vi "Ex_Inst_Write LabVIEW Measurement File.vi"(0 "Signals":dynamicdata(waveform), 2 "Enable":bool=TRUE, 5 "error in (no error)":errorcluster, 8 "Filename":path, 10 "Comment":string, 11 "DAQmx Task":refnum<k21>) -> (16 "Filename Out":path, 17 "Saving Data":bool, 19 "error out":errorcluster)   [LabVIEW 2020]
doc: "Writes data to text-based measurement files (.lvm), binary measurement files (.tdm or .tdms), or Microsoft Excel files (.xlsx)."
uses:
  <vilib>/express/express shared/ExFile.llb/ex_FileFormats.ctl
  <vilib>/express/express shared/ExFile.llb/ex_userDefProperty.ctl
  <vilib>/express/express shared/ex_EditUserDefinedProperties/usiDataType.ctl
  <vilib>/express/express shared/ExFile.llb/ex_propertySource.ctl
panel:
  in  "Live values":variant[](array[variant])
  in  "new_file":bool
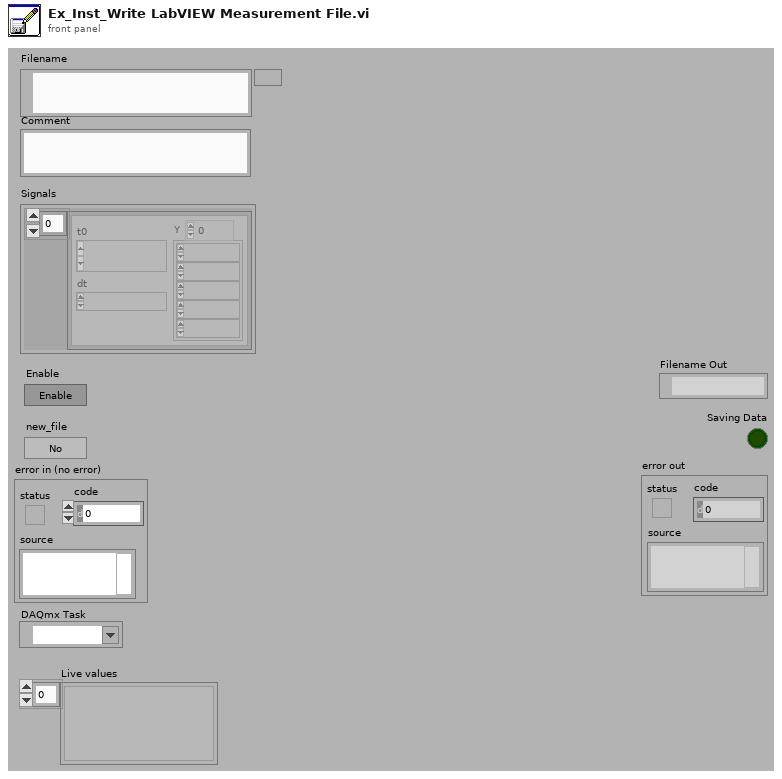
[diagram p1: front panel]
types:
  T1 = cluster{"Boolean":bool, "Timestamp format":string}
  T2 = typedef "ex_FileFormats.ctl" = enum32{"lvm", "tdm", "tdms", "xlsx"}
  T3 = typedef "ex_userDefProperty.ctl" = cluster{"Name":string, "Object type":string, "usiDataType":T4, "propertySourceType":T5, "propertySource":string, "Value":variant, "ID":i32, "use def name":bool, "Source":string, "Built-in Prop":bool, "Attribute Type Enum":string[]}
  T4 = typedef "usiDataType.ctl" = enum16{"eNoTypeUsi", "eInt8Usi", "eInt16Usi", "eInt32Usi", "eInt64Usi", "eUInt8Usi", "eUInt16Usi", "eUInt32Usi", "eUInt64Usi", "eFloat32Usi", "eFloat64Usi", "- 0", "- 1", "- 2", "- 3", "- 4", "- 5", "- 6", "- 7", "- 8", "- 9", "eString8Usi", "eString16Usi", "eStringUsi", "eEnumUsi", "- 10", "- 11", "- 12", "- 13", "- 14", "eTimeUsi", "- 15", "- 16", "- 17", "- 18", "- 19", "- 20", "- 21", "- 22", "- 23", "eInstanceUsi", "eStoreUsi"}
  T5 = typedef "ex_propertySource.ctl" = enum16{"Manual", "System", "DAQmx Channel", "Terminal", "Ignore"}
  T6 = cluster{"Description":string, "Configure User Def Prop In":cluster{"user-def properties in":T3[], "selected nodes in":string[]}, "Comment":string, "DAQmx Task":string, "Live values":variant[]}
  T7 = cluster{"user-def properties in":T3[], "selected nodes in":string[]}
  T8 = enum32{"overwrite", "overwrite & backup", "append", "next avail"}
  T9 = enum16{"overwrite", "overwrite & backup", "next avail"}
  T10 = cluster{"new_file_iter":bool, "new_file_#iter":i32}
  T11 = cluster{"new_file_samples":bool, "new_file_#samples":i32}
  T12 = cluster{"new_file_size":bool, "new_file_max_size":i32}
  T13 = cluster{"new_file_elaps_time":bool, "max_elapsed_seconds":i32}
  T14 = cluster{"new_file_daily":bool, "new_file_timeofday":i32}
  T15 = cluster{cluster{"new_file_iter":bool, "new_file_#iter":i32}, cluster{"new_file_samples":bool, "new_file_#samples":i32}, cluster{"new_file_size":bool, "new_file_max_size":i32}, cluster{"new_file_elaps_time":bool, "max_elapsed_seconds":i32}, cluster{"new_file_daily":bool, "new_file_timeofday":i32}}
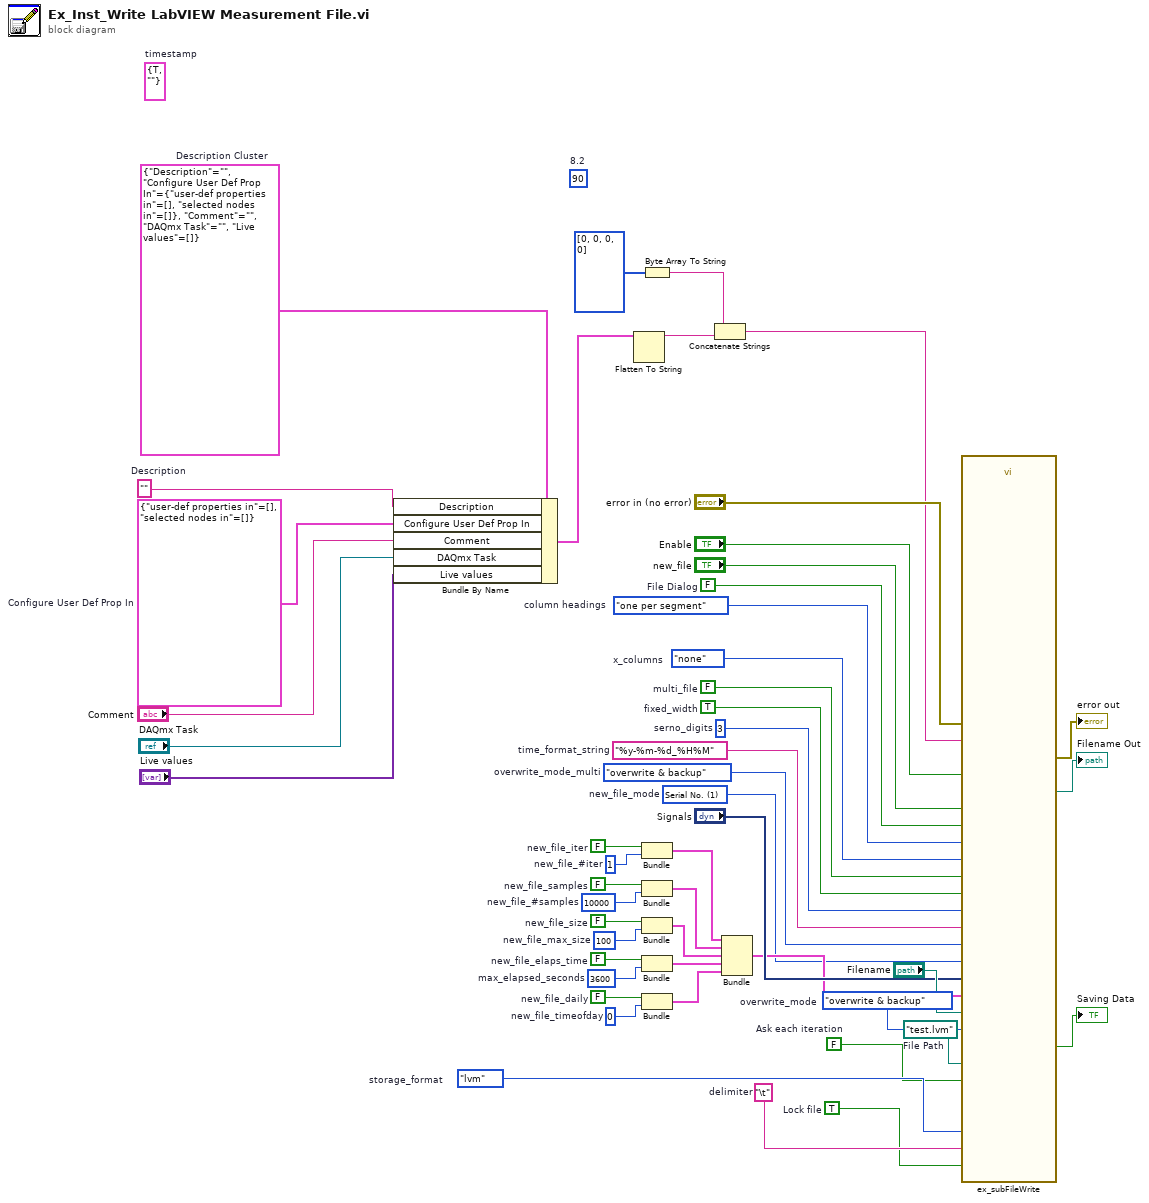
[diagram p0: block diagram]
diagram:
  (unwired) T1 {"Boolean"=TRUE, "Timestamp format"=""}  # timestamp
  (unwired) 90  # 8.2
  w18 = ex_FileFormats."lvm"  # storage_format
  w30 = T6 {"Description"="", "Configure User Def Prop In"={"user-def properties in"=[], "selected nodes in"=[]}, "Comment"="", "DAQmx Task"="", "Live values"=[]}  # Description Cluster
  w28 = TRUE  # Lock file
  w21 = T7 {"user-def properties in"=[], "selected nodes in"=[]}  # Configure User Def Prop In
  w22 = ""  # Description
  w31 = "\t"  # delimiter
  w8 = T8."overwrite & backup"  # overwrite_mode
  w13 = enum32{"none", "one", "multiple"}."none"  # x_columns
  w32 = enum32{"one per segment", "once", "none"}."one per segment"  # column headings
  w10 = FALSE  # Ask each iteration
  w4 = T9."overwrite & backup"  # overwrite_mode_multi
  w7 = u16 1 items=["Date & Time", "Serial No.", "Both"]  # new_file_mode
  w6 = "%y-%m-%d_%H%M"  # time_format_string
  w5 = TRUE  # fixed_width
  w3 = 3  # serno_digits
  w42 = 0  # new_file_timeofday
  w43 = FALSE  # new_file_daily
  w35 = 3600  # max_elapsed_seconds
  w44 = FALSE  # new_file_elaps_time
  w45 = 100  # new_file_max_size
  w46 = FALSE  # new_file_size
  w47 = 10000  # new_file_#samples
  w49 = 1  # new_file_#iter
  w48 = FALSE  # new_file_samples
  w50 = FALSE  # new_file_iter
  w16 = FALSE  # multi_file
  w14 = FALSE  # File Dialog
  w2 = path "test.lvm"  # File Path
  n1 = Bundle By Name(cluster=w30, "Description"=w22, "Configure User Def Prop In"=w21, "Comment"="Comment", "DAQmx Task"="DAQmx Task", "Live values"="Live values") -> (w27:T6)
  n2 = Flatten To String(anything=w27) -> (data string=w24:string)  [unwired: 1 in, 4 out]
  n3 = Byte Array To String(unsigned byte array=u8[] [0, 0, 0, 0]) -> (string=w23:string)
  n4 = Bundle("new_file_iter"=w50, "new_file_#iter"=w49) -> (w41:T10)  [unwired: 1 out]
  n5 = Bundle("new_file_samples"=w48, "new_file_#samples"=w47) -> (w40:T11)  [unwired: 1 out]
  n6 = Bundle("new_file_size"=w46, "new_file_max_size"=w45) -> (w37:T12)  [unwired: 1 out]
  n7 = Bundle("new_file_elaps_time"=w44, "max_elapsed_seconds"=w35) -> (w39:T13)  [unwired: 1 out]
  n8 = Bundle("new_file_daily"=w43, "new_file_timeofday"=w42) -> (w38:T14)  [unwired: 1 out]
  n9 = Concatenate Strings(w23, w24) -> (w25:string)
  n10 = Bundle(w41, w40, w37, w39, w38) -> (w9:T15)  [unwired: 1 out]
  n11 = call <vilib>:"ex_subFileWrite.vi"("Signals"="Signals", "error in (no error)"="error in (no error)", "Comment"=w25, "Enable"="Enable", "new_file"="new_file", "File Path in"="Filename", "File Dialog"=w14, "column headings"=w32, "x_columns"=w13, "multi_file"=w16, "fixed_width"=w5, "serno_digits"=w3, "time_format_string"=w6, "overwrite_mode_multi"=w4, "new_file_mode"=w7, "overwrite_mode"=w8, "new file options"=w9, "delimiter"=w31, "Static File Path in"=w2, "Lock file"=w28, "storage_format"=w18, "Ask each iteration"=w10) -> ("error out"=→"error out":errorcluster, "File Path out"=→"Filename Out":path, "Saving Data"=→"Saving Data":bool)  [unwired: 3 in]
